vi "ProcLambda.vi"(2 "Body":u8[](array[numeric]), 3 "Length":u16) -> (0 "Lambda":dbl format="%.2f", 1 "Error":u32)   [LabVIEW 2016]
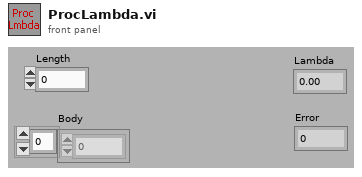
[diagram p1: front panel]
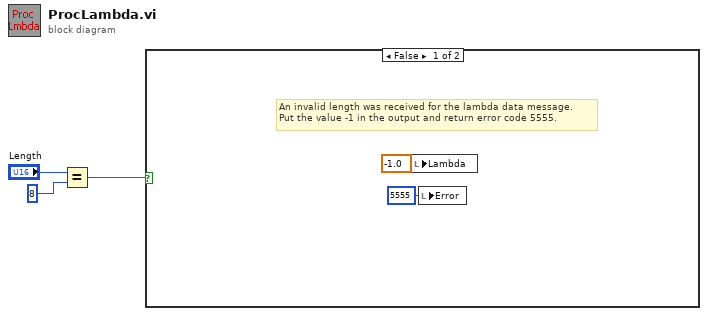
[diagram p0: block diagram]
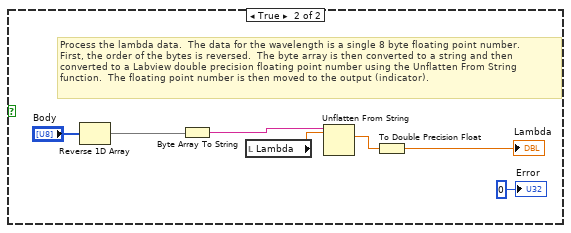
[diagram p2: hidden frame]
diagram:
  n1 = Equal?(x="Length", y=u16 8) -> (x = y?=w1:bool)
  n2 = case shown="False" w1 {
    frame False {
      # "An invalid length was received for the lambda data message.\nPut the value -1 in the output and return error code 5555."
      n3 = local write "Lambda"(-1.0 ("Lambda")) -> ()
      n4 = local write "Error"(u32 5555 ("Error")) -> ()
    }
    frame True {
      # "Process the lambda data.  The data for the wavelength is a single 8 byte floating point number.\nFirst, the order of the bytes is reversed.  The byte array is then converted to a string and then\nconverted to a Labview double precision floating point number using the Unflatten From String\nfunction.  The floating point number is then moved to the output (indicator)."
      n5 = Reverse 1D Array(array="Body") -> (reversed array=w7:u8[])
      n6 = Byte Array To String(unsigned byte array=w7) -> (string=w10:string)
      n7 = local read "Lambda"() -> (w9:dbl)
      n8 = Unflatten From String(type=w9, binary string=w10) -> (value=w11:dbl)  [unwired: 3 in, 2 out]
      n9 = To Double Precision Float(number=w11) -> (double precision float=→"Lambda":dbl)
      "Error" <- u32 0 ("Error")
    }
  }
